vi "upload.sign_part.vi"(6 "Part Number":i32, 8 "error in":errorcluster, 11 "Multipart Upload in":refnum<class "Multipart Upload.lvclass">) -> (0 "error out":errorcluster, 3 "Multipart Upload out":refnum<class "Multipart Upload.lvclass">)   [LabVIEW 2020, in "Multipart Upload.lvclass"]
doc: "Signs an upload request for a single part. Returns a URL that will execute the upload without further authentication.\n\nThe Part Number must be greater than 0."
uses:
  Multipart Upload.lvclass
  Multipart Upload.lvclass/Multipart Upload.ctl
  8b3dcdab-c30a-41f7-882b-0fd92512159b.vi
  nominal_client.get.vi
  <vilib>/JDP Science/JSONtext/JSON text to Variant.vi
  Nominal Client/Nominal Client.lvclass
  <vilib>/JDP Science/JSONtext/LVClass Serializer/JSONtext LVClass Serializer.lvclass
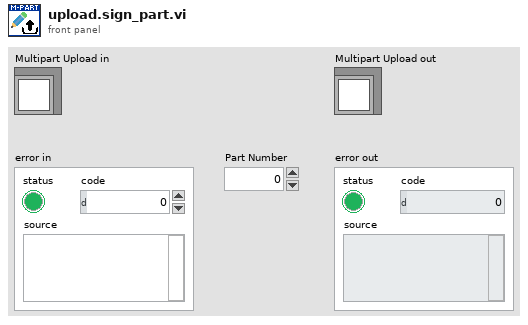
[diagram p1: front panel]
types:
  T1 = cluster{"url":string, "headers":map{string, string}}
  T2 = map{i32, cluster{"url":string, "headers":map{string, string}}}
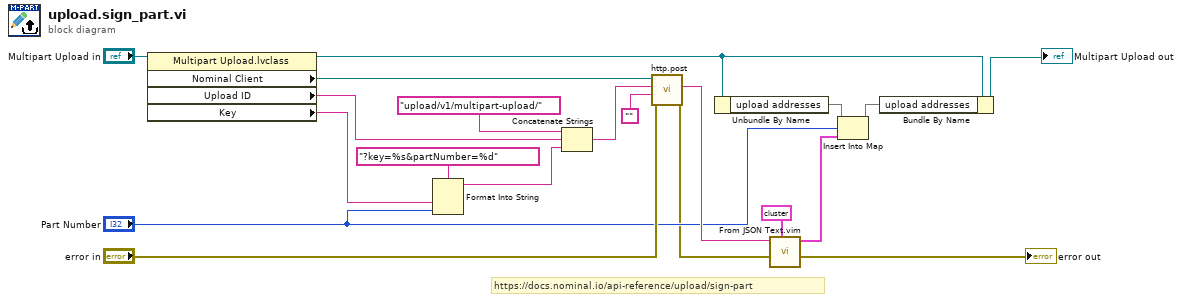
[diagram p0: block diagram]
diagram:
  # "https://docs.nominal.io/api-reference/upload/sign-part"
  n1 = property class="Multipart Upload.lvclass"(reference="Multipart Upload in") -> (reference out=w6:refnum<class "Multipart Upload.lvclass">, "Nominal Client"=w10:refnum<class "Nominal Client.lvclass">, "Upload ID"=w13:string, "Key"=w12:string)  [unwired: 1 in, 1 out]
  n2 = Format Into String(format string="?key=%s&partNumber=%d" ("Path"), w12, "Part Number") -> (resulting string=w15:string)  [unwired: 2 in, 1 out]
  n3 = Concatenate Strings("upload/v1/multipart-upload/" ("Path"), w13, w15) -> (w18:string)
  n4 = call "http.post.vi"("error in"="error in", "Request body"="", "Path"=w18, "Nominal Client in"=w10) -> ("error out"=w3:errorcluster, "Response"=w20:string)  [unwired: 5 in, 1 out]
  n5 = Unbundle By Name(w6) -> ("upload addresses"=w9:T2)
  n6 = call "From JSON Text.vim"("Data Type and Default Value"=T1 {"url"="", "headers"={}} ("addresses"), "error in (no error)"=w3, "JSON"=w20) -> ("error out"=→"error out":errorcluster, "Data out"=w8:T1)  [unwired: 7 in]
  n7 = Insert Into Map(map in=w9, key="Part Number", value=w8) -> (map out=w4:T2)  [unwired: 2 out]
  n8 = Bundle By Name(cluster=w6, "upload addresses"=w4) -> (→"Multipart Upload out":refnum<class "Multipart Upload.lvclass">)
